vi "inputView.vi"(10 "UserEvents in":refnum<class "UserEvents.lvclass">) -> ()   [LabVIEW 2013, in "ILCBTViews.lvlib"]
uses:
  ILCBTViews.lvlib
  UserEvents/UserEvents.lvclass
  UserEvents/UserEvents.lvclass/UserEvents.ctl
  Typedefs/StateSelector.ctl
  Typedefs/ILCBTTypedefs.lvlib
types:
  T1 = typedef "ILCBTTypedefs.lvlib/PubDataEvents.ctl" = cluster{"State":refnum<user-event>, "ErrorCode":refnum<user-event>, "OutputData":refnum<user-event>, "LogPath":refnum<user-event>}
  T2 = cluster{"Event Registration Refnum":refnum<event-registration>}
  T3 = typedef "ILCBTTypedefs.lvlib/StateSelector.ctl" = enum16{"EnabledState", "FaultState", "OffState", "StandbyState"}
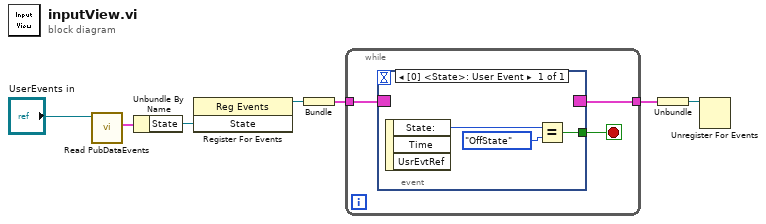
[diagram p0: block diagram]
diagram:
  n1 = call "Read PubDataEvents.vi"("UserEvents in"="UserEvents in") -> ("PubDataEvents"=w7:T1)  [unwired: 9 in, 1 out]
  n2 = Unbundle By Name(w7) -> ("State"=w6:refnum<user-event>)
  n3 = register-events(w6) -> (reference out=w5:refnum<event-registration>)  [unwired: 2 in, 1 out]
  n4 = Bundle("Event Registration Refnum"=w5) -> (w3:T2)  [unwired: 1 in]
  n5 = while {
    tunnel: w3 -> [w10]
    tunnel: [w8] -> w2
    stop <- w9 stop-if-true
    n6 = event shown="[0] <State>: User Event" {
      selector: w10 -> [_]
      dyn-events: [_] -> w8
      timeout: _ -> [_]
      tunnel: [w12] -> w9
      event User Event {
        n7 = event-data() -> ("State:"=w11:T3)  [unwired: 1 in, 2 out]
        n8 = Equal?(x=w11, y=StateSelector."OffState" ("State:")) -> (x = y?=w12:bool)
      }
    }
  }
  n9 = Unbundle(w2) -> ("Event Registration Refnum"=w1:refnum<event-registration>)
  n10 = Unregister For Events(event registration refnum=w1) -> ()  [unwired: 1 in, 1 out]
